vi "Acquire Array of Waveforms (simulated).vi"(8 "error in (no error)":errorcluster, 11 "# of waveforms to create":i32=3) -> (0 "error out":errorcluster, 3 "Array of Waveforms":waveform(dbl)[](array[waveform]))   [LabVIEW 2020]
doc: "Creates an array of waveforms. The waveform values are randomly generated."
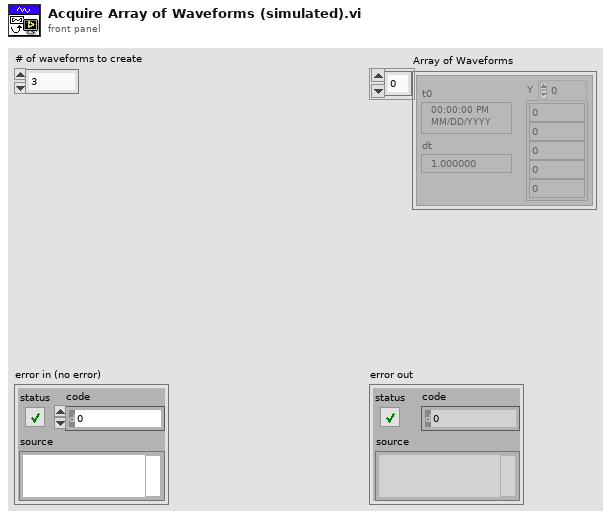
[diagram p1: front panel]
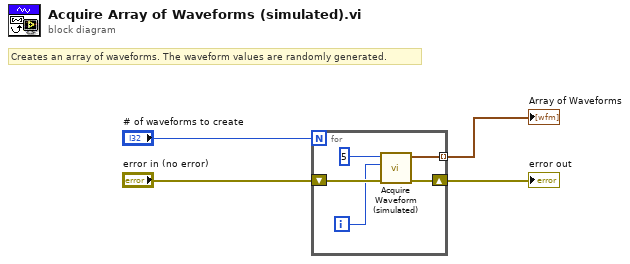
[diagram p0: block diagram]
diagram:
  # "Creates an array of waveforms. The waveform values are randomly generated."
  n1 = for {
    N: "# of waveforms to create" -> [_]
    tunnel: [w8] -> w3 mode=indexing
    shift-right: [w6] -> w1
    shift-left: "error in (no error)" -> [w7]
    i -> [w5]
    n2 = call "Acquire Waveform (simulated).vi"("error in (no error)"=w7, "channel #"=w5, "# points"=5) -> ("error out"=w6:errorcluster, "waveform output"=w8:waveform(dbl))  [unwired: 7 in]
  }
  "Array of Waveforms" <- w3
  "error out" <- w1
